vi "Close HVPS.vi"(8 "error in":errorcluster, 11 "DAQ HVPS in":refnum<class "DAQ HVPS.lvclass">) -> (0 "error out":errorcluster, 3 "DAQ HVPS out":refnum<class "DAQ HVPS.lvclass">)   [LabVIEW 2014, in "DAQ HVPS.lvclass"]
doc: "Use this method to gracefully close connections and destroy references."
uses:
  Session Based/DAQ/DAQ HVPS.lvclass
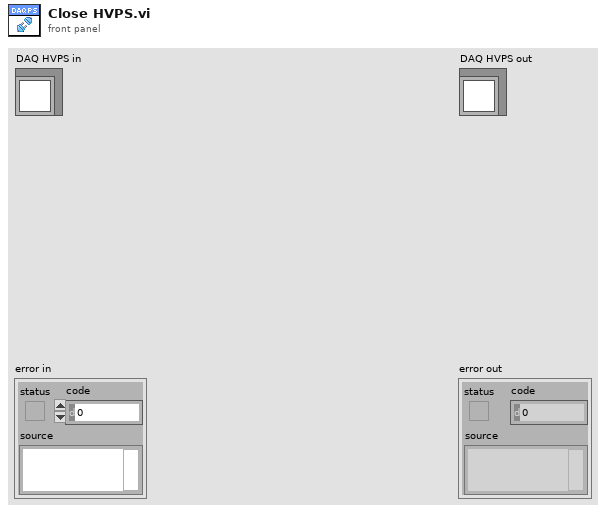
[diagram p1: front panel]
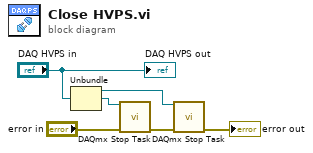
[diagram p0: block diagram]
diagram:
  n1 = Unbundle("DAQ HVPS in") -> (w4:refnum<k21>, w5:refnum<k21>)  [unwired: 1 out]
  n2 = call <vilib>:"DAQmx Stop Task.vi"("task/channels in"=w5, "error in"="error in") -> ("error out"=w3:errorcluster)  [unwired: 12 in, 1 out]
  n3 = call <vilib>:"DAQmx Stop Task.vi"("task/channels in"=w4, "error in"=w3) -> ("error out"=→"error out":errorcluster)  [unwired: 12 in, 1 out]
  "DAQ HVPS out" <- "DAQ HVPS in"
